vi "seriellFIFORTTest.vi"() -> ()   [LabVIEW 2010]
uses:
  <vilib>/rvi/interface/nirviReadWriteControl/nirviReadWriteControl.xnode
  C:/Users/HAGAR-IV/Desktop/Zeugs/markus/version feb 2012/FPGA Bitfiles/pertrasgcfpga2_FPGATarget_FPGA-Programm-10_16368CB6.lvbitx
  C:/Users/HAGAR-IV/Desktop/Zeugs/Johnny/pertrasgc fpga/FPGA-Programm-10-14.vi
  <vilib>/rvi/interface/nirviCloseFPGA/nirviCloseFPGA.xnode
  NiFpgaLv.dll
  <vilib>/Utility/error.llb/Error Cluster From Error Code.vi
  <vilib>/rvi/errors/niLvFpgaWhatHappensToTopLevelVI.ctl
  <vilib>/rvi/interface/common/niFpgaNodeNameForErrorReporting.ctl
  <vilib>/rvi/errors/niLvFpgaAdjustHostInterfaceError.vi
  <vilib>/FPGAPlugInAG/cRIO-9114/niLvFpga_Close_cRIO-9114.vi
panel:
  in  "Stopp":bool
  in  "AnzahlHorst":i32[](array[numeric])
  out "HorstMW":dbl[](array[numeric])
  in  "HorstSPVorwort":string[](array[string])
  in  "HorstAbfragen":string[](array[string])
  in  "HorstSP":dbl[](array[numeric])
  in  "HorstSP0":dbl[](array[numeric])
  in  "SkalierungsfaktorHorst":dbl[](array[numeric])
  in  "VorwortHorst":string[](array[string])
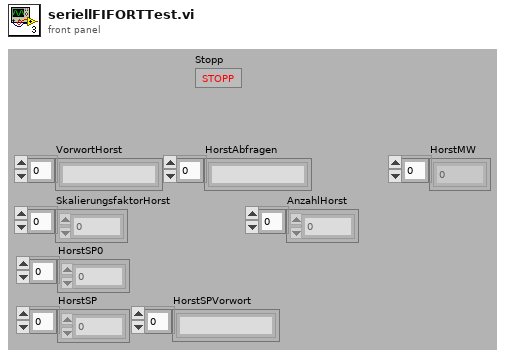
[diagram p1: front panel]
types:
  T1 = cluster{string[], string[], string[], dbl[], dbl[], dbl[]}
  T2 = cluster{"Befehle1":string[], "Befehle2":string[], "Befehle3":string[]}
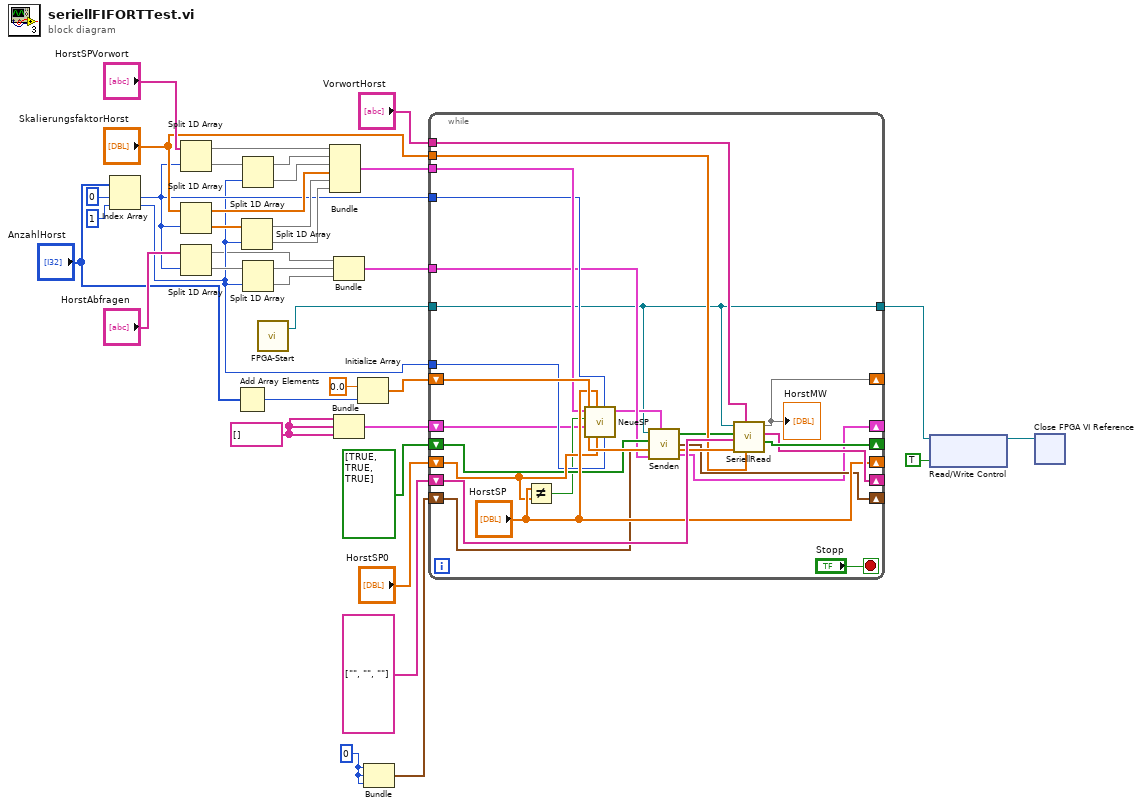
[diagram p0: block diagram]
diagram:
  w12 = 0
  w10 = string[] []
  n1 = Index Array(array="AnzahlHorst", index #1=0 ("Index"), index #2=1 ("Index")) -> (element #1=w19:i32, element #2=w17:i32)
  n2 = Split 1D Array(array="HorstSPVorwort", index=w19) -> (first subarray=w27:string[], second subarray=w30:string[])
  n3 = Split 1D Array(array="SkalierungsfaktorHorst", index=w19) -> (first subarray=w24:dbl[], second subarray=w28:dbl[])
  n4 = Split 1D Array(array="HorstAbfragen", index=w19) -> (first subarray=w16:string[], second subarray=w18:string[])
  n5 = Add Array Elements(numeric array="AnzahlHorst") -> (sum=w7:i32)
  n6 = Split 1D Array(array=w28, index=w17) -> (first subarray=w23:dbl[], second subarray=w22:dbl[])
  n7 = Split 1D Array(array=w30, index=w17) -> (first subarray=w26:string[], second subarray=w25:string[])
  n8 = Split 1D Array(array=w18, index=w17) -> (first subarray=w15:string[], second subarray=w14:string[])
  n9 = call "FPGA-Start.vi"() -> ("FPGA VI Reference Out"=w4:refnum<k20>)  [unwired: 2 in, 1 out]
  n10 = Bundle(w27, w26, w25, w24, w23, w22) -> (w21:T1)  [unwired: 1 in]
  n11 = Bundle(w16, w15, w14) -> (w13:cluster{string[], string[], string[]})  [unwired: 1 in]
  n12 = Bundle(w10, w10, w10) -> (w9:cluster{string[], string[], string[]})  [unwired: 1 in]
  n13 = Initialize Array(0.0 ("Element"), w7) -> (w5:dbl[])
  n14 = Bundle(w12, w12, w12) -> (w11:cluster{i32, i32, i32})  [unwired: 1 in]
  n15 = while {
    shift-right: [w60] -> _
    shift-left: bool[] [TRUE, TRUE, TRUE] -> [w47]
    shift-right: ["HorstSP"] -> _
    shift-left: "HorstSP0" -> [w51]
    tunnel: w4 -> [w38]
    shift-right: [w58] -> _
    shift-left: string[] ["", "", ""] -> [w59]
    shift-right: [w57] -> _
    shift-left: w5 -> [w56]
    tunnel: "VorwortHorst" -> [w55]
    tunnel: "SkalierungsfaktorHorst" -> [w54]
    shift-right: [w40] -> _
    shift-left: w9 -> [w42]
    tunnel: w19 -> [w49]
    tunnel: w17 -> [w50]
    tunnel: w21 -> [w52]
    tunnel: w13 -> [w45]
    shift-right: [w44] -> _
    shift-left: w11 -> [w46]
    tunnel: [w38] -> w3
    stop <- "Stopp" stop-if-true
    n16 = Not Equal?(x="HorstSP", y=w51) -> (x != y?=w43:bool)
    n17 = call "NeueSP.vi"("Anzahl2"=w50, "Anzahl1"=w49, "AlteSP"=w51, 7:"NeueSP"="HorstSP", "BefehleCluster"=w42, 10:"NeueSP"=w43, "ClusterFest"=w52) -> ("BefehleCluster"=w41:T2)  [unwired: 4 in]
    n18 = call "Senden.vi"("FPGA VI Reference In"=w38, "BefehlsCluster"=w41, "Senden?"=w47, "Abfragenr.Cluster"=w46, "AbfragenCluster"=w45) -> ("Senden?"=w48:bool[], "Abfragenr.Cluster"=w44:cluster{i32, i32, i32}, "BefehlsCluster"=w40:T2)  [unwired: 1 in]
    n19 = call "SeriellRead.vi"("SkalierungsfaktorHorst"=w54, "VorwortHorst"=w55, 8:w56, "Zwischenspeicher"=w59, "Senden?"=w48, "FPGA VI Reference In"=w38) -> ("Senden?"=w60:bool[], "Zwischenspeicher"=w58:string[], 3:w57)  [unwired: 3 in]
    "HorstMW" <- w57
  }
  n20 = xnode "Read/Write Control"("FPGA VI Reference In"=w3, "global stop"=TRUE) -> ("FPGA VI Reference Out"=w1:refnum<k20>)  [unwired: 1 in, 1 out]
  n21 = xnode "Close FPGA VI Reference"("FPGA VI Reference In"=w1) -> ()  [unwired: 1 in, 1 out]
